vi "打包.vi"(1 "总内容":string, 2 "分包大小":i32=1) -> (0 "分包数组":string[](array[string]))   [LabVIEW 2016, in "数据传输系统-05.lvlib" / "自动更新.lvlib" / "TCP文件传输系统.lvlib" / "TCP发送文件.lvlib"]
panel:
  out "总内容长度":i32
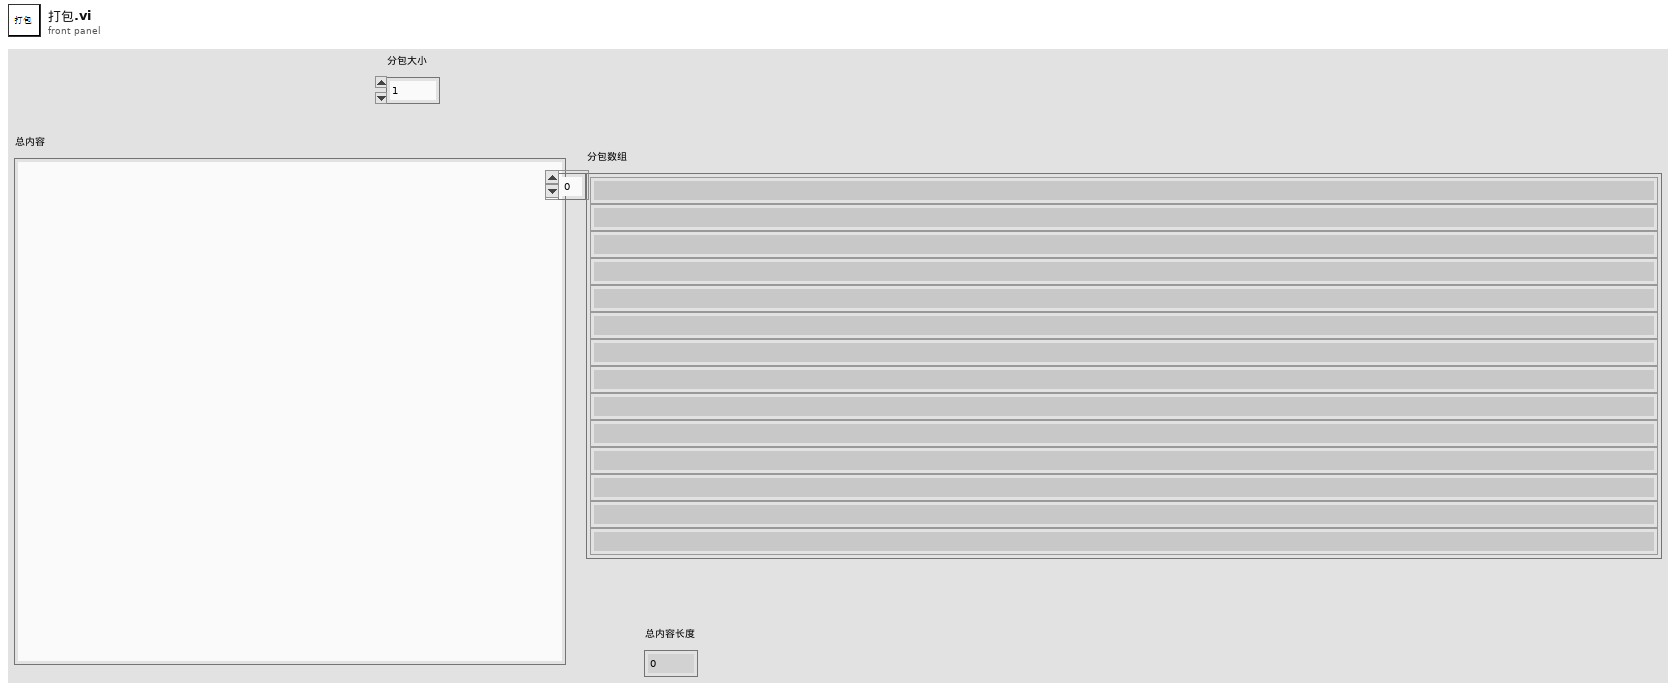
[diagram p1: front panel]
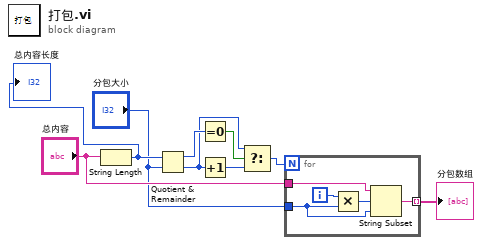
[diagram p0: block diagram]
diagram:
  n1 = String Length(string="总内容") -> (length=w9:i32)
  "总内容长度" <- w9
  n2 = Quotient & Remainder(x=w9, y="分包大小") -> (x-y*floor(x/y)=w6:i32, floor(x/y)=w3:i32)
  n3 = Equal To 0?(x=w6) -> (x = 0?=w5:bool)
  n4 = Increment(x=w3) -> (x+1=w4:i32)
  n5 = Select(t=w3, s=w5, f=w4) -> (s? t:f=w2:i32)
  n6 = for {
    N: w2 -> [_]
    tunnel: "总内容" -> [w14]
    tunnel: "分包大小" -> [w11]
    tunnel: [w10] -> w1 mode=indexing
    i -> [w13]
    n7 = Multiply(x=w13, y=w11) -> (x*y=w12:i32)
    n8 = String Subset(string=w14, offset (0)=w12, length (rest)=w11) -> (substring=w10:string)
  }
  "分包数组" <- w1
